vi "Write External Payload.vi"(8 "error in (no error)":errorcluster, 9 "Timeout (ms)":i32, 10 "U8 With Header in":u8[](array[numeric]), 11 "CIFFIFO in":refnum<class "CIF_NIChn_Fifo_U8.lvclass">) -> (0 "error out":errorcluster, 1 "timed out?":bool, 2 "U8 With Header out":u8[](array[numeric]), 3 "CIFFIFO out":refnum<class "CIF_NIChn_Fifo_U8.lvclass">)   [LabVIEW 2021, in "CIF_NIChn_Fifo_U8.lvclass"]
uses:
  CIF_NIChn_Fifo_U8.lvclass
  CIF_NIChn_Fifo_U8.lvclass/CIF_NIChn_Fifo_U8.ctl
  CIFChannels/CIFChannels.lvclass
  ChannelCommon/ChannelCommon.lvlib
  ChannelCommon/typedef/TimeStamps.ctl
  D:/dev/Packages/Channel_Manager/src/CIF_NIChn/NIChn/CIF_NIChn.lvclass
  D:/dev/Packages/Channel_Manager/src/CIFChannels/CIFChannels.lvclass
  D:/dev/Packages/Channel_Manager/src/CIF_NIChn/FIFO_U8 - Copy/CIF_NIChn_Fifo_U8.lvclass
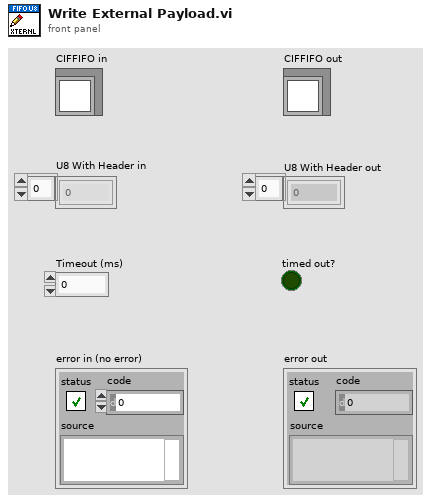
[diagram p1: front panel]
types:
  T1 = typedef "ChannelCommon.lvlib/TimeStamps.ctl" = cluster{"ClockID":u8, "T0":i64, "T_Out":i64}
  T2 = typedef "ChannelCommon.lvlib/FIFO Header.ctl" = cluster{"Length":u64, "T0":i64, "T_Out":i64, "T_Tx":i64, "Ctr":u64, "ClockID":u8}
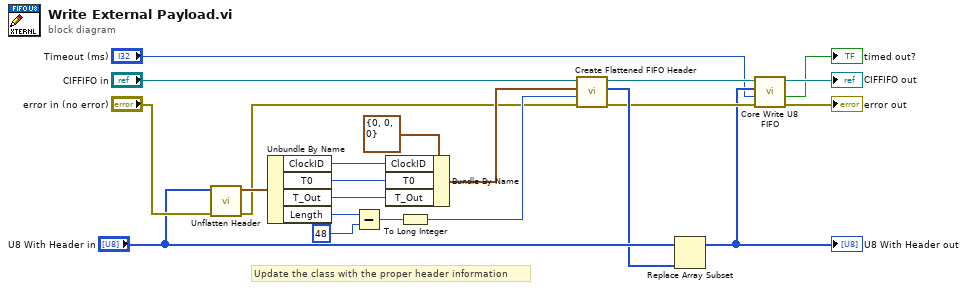
[diagram p0: block diagram]
diagram:
  # "Update the class with the proper header information"
  n1 = call "Unflatten Header.vi"("error in (no error)"="error in (no error)", "Flattened Data in"="U8 With Header in") -> ("error out"=w10:errorcluster, "Header out"=w21:T2)  [unwired: 7 in, 1 out]
  n2 = Unbundle By Name(w21) -> ("ClockID"=w12:u8, "T0"=w13:i64, "T_Out"=w14:i64, "Length"=w20:u64)
  n3 = Subtract(x=w20, y=u64 48) -> (x-y=w18:u64)
  n4 = Bundle By Name(cluster=T1 {"ClockID"=0, "T0"=0, "T_Out"=0} ("FIFO Timestamps"), "ClockID"=w12, "T0"=w13, "T_Out"=w14) -> (w15:T1)
  n5 = To Long Integer(number=w18) -> (32bit integer=w17:i32)
  n6 = call "Create Flattened FIFO Header.vi"("error in (no error)"=w10, "Data Length"=w17, "FIFO Timestamps"=w15, "CIFChannels in"="CIFFIFO in") -> ("error out"=w6:errorcluster, "Flattened FIFO Header"=w8:u8[], "CIFChannels out"=w7:refnum<class "CIF_NIChn_Fifo_U8.lvclass">)  [unwired: 5 in]
  n7 = Replace Array Subset(array="U8 With Header in", new element=w8) -> (w2:u8[])  [unwired: 1 in]
  "U8 With Header out" <- w2
  n8 = call "Core Write U8 FIFO.vi"("error in (no error)"=w6, "Timeout (ms)"="Timeout (ms)", "U8 With Header in"=w2, "CIFFIFO in"=w7) -> ("error out"=→"error out":errorcluster, "timed out?"=→"timed out?":bool, "CIFFIFO out"=→"CIFFIFO out":refnum<class "CIF_NIChn_Fifo_U8.lvclass">)  [unwired: 4 in, 1 out]
